vi "Start Polling.vi"(8 "error in (no error)":errorcluster, 11 "PID Loop in":refnum<class "PID Loop.lvclass">) -> (0 "error out":errorcluster, 3 "PID Loop out":refnum<class "PID Loop.lvclass">)   [LabVIEW 2024, in "PID Loop.lvlib" / "PID Loop.lvclass"]
uses:
  PID Loop.lvclass
  PID Loop.lvclass/PID Loop.ctl
  OOQMH/OOQMH/OOQMH.lvclass
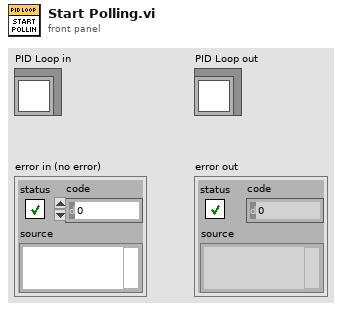
[diagram p1: front panel]
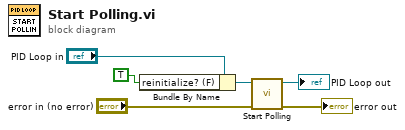
[diagram p0: block diagram]
diagram:
  n1 = Bundle By Name(cluster="PID Loop in", "reinitialize? (F)"=TRUE) -> (w1:refnum<class "PID Loop.lvclass">)
  n2 = call-parent "Start Polling.vi"("error in (no error)"="error in (no error)", "OOQMH in"=w1) -> ("error out"=→"error out":errorcluster, "OOQMH out"=→"PID Loop out":refnum<class "PID Loop.lvclass">)  [unwired: 8 in]
